vi "Differential Pressure Release Valve Test DAA.vi"(8 "error in (no error)":errorcluster, 10 "Model in":refnum<class "Model.lvclass">, 11 "Test Actuator State in":refnum<class "Test Actuator State.lvclass">) -> (0 "error out":errorcluster, 1 "Pass":bool, 2 "Model out":refnum<class "Model.lvclass">, 3 "Test Actuator State out":refnum<class "Test Actuator State.lvclass">)   [LabVIEW 2016, in "Test Actuator State.lvclass"]
uses:
  Test Actuator State.lvclass
  Model/Model/Model.lvclass
  Model/Model/Model.lvclass/Model.ctl
  Typedefs/ActuatorSetPoints.ctl
  <vilib>/Platform/TimedLoop/XDataNode/timing_clust.ctl
  <vilib>/Platform/TimedLoop/XDataNode/nitl_modes.ctl
  <vilib>/Platform/TimedLoop/XDataNode/wakeup.ctl
  <vilib>/platform/TimedLoop/XDataNode/XDataNode.xnode
  Typedefs/FAMT Typedefs.lvlib
  <vilib>/Platform/TimedLoop/XDataNode/XDNodeRunTimeDep.lvlib
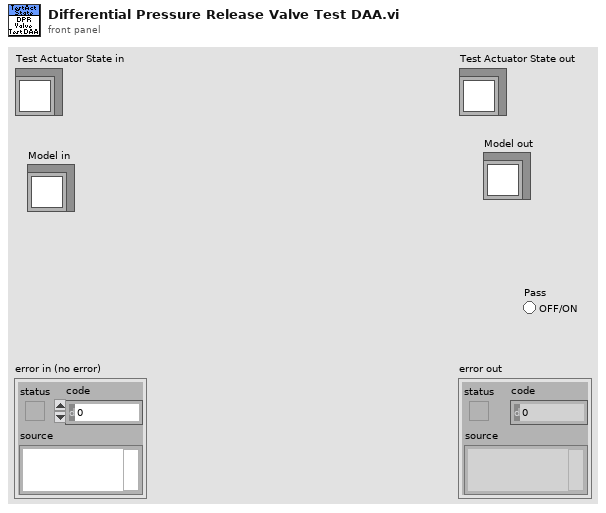
[diagram p1: front panel]
types:
  T1 = typedef "FAMT Typedefs.lvlib/DifferentialPressureReleaseValveTestSettings.ctl" = cluster{"Max Over Force (N)":dbl, "Process Time (s)":dbl, "Sample Time (s)":dbl}
  T2 = typedef "FAMT Typedefs.lvlib/ForcePair.ctl" = cluster{"Axial Force":dbl, "Lateral Force":dbl}
  T3 = typedef "FAMT Typedefs.lvlib/FullForceScanSettings.ctl" = cluster{"Force Tolerance (N)":dbl, "DAA Force Set Points":T2[], "Process Time (s)":dbl, "Sample Time (s)":dbl, "SAA Force Set Points":T2[]}
  T4 = cluster{"Top Left":T2, "Top Right":T2, "Bottom Right":T2, "Bottom Left":T2}
  T5 = typedef "FAMT Typedefs.lvlib/ActuatorSetPoints.ctl" = cluster{"Axial Force":dbl, "Lateral Force":dbl, "FC1 Force":dbl, "FC2 Force":dbl}
  T6 = typedef "XDNodeRunTimeDep.lvlib/timing_clust.ctl" = cluster{"Expected End [f-1]":u64, "Actual End [f-1]":u64, "Finished Late? [f-1]":bool, "Expected End [i-1]":u64, "Actual End [i-1]":u64, "Finished Late? [i-1]":bool, "Expected Start [i]":u64, "Actual Start [i]":u64, "Expected Start [f]":u64, "Actual Start [f]":u64, "Source Name":string, "Structure Name":string, "Period":i64, "Deadline":i64, "Offset":i64, "Start":i64, "Priority":i32, "Timeout":i32, "Mode":T7, "Wakeup Reason":T8, "Error":errorcluster, "Source Type":string, "Secondary Source Type":string, "Global End Time":u64, "Global Start Time":u64, "Frame Duration":u64, "Iteration Duration":u64, "Assigned CPU":i32, "I/O Scan Engine Mode":u32}
  T7 = typedef "XDNodeRunTimeDep.lvlib/nitl_modes.ctl" = enum32{"No Change", "Process missed periods, maintain original phase", "Discard missed periods, maintain original phase", "Process missed periods, ignore original phase", "Discard missed periods, ignore original phase"}
  T8 = typedef "XDNodeRunTimeDep.lvlib/wakeup.ctl" = enum32{"Normal", "Aborted", "Asynchronous wakeup", "Timing source error", "Timed loop error", "Timeout"}
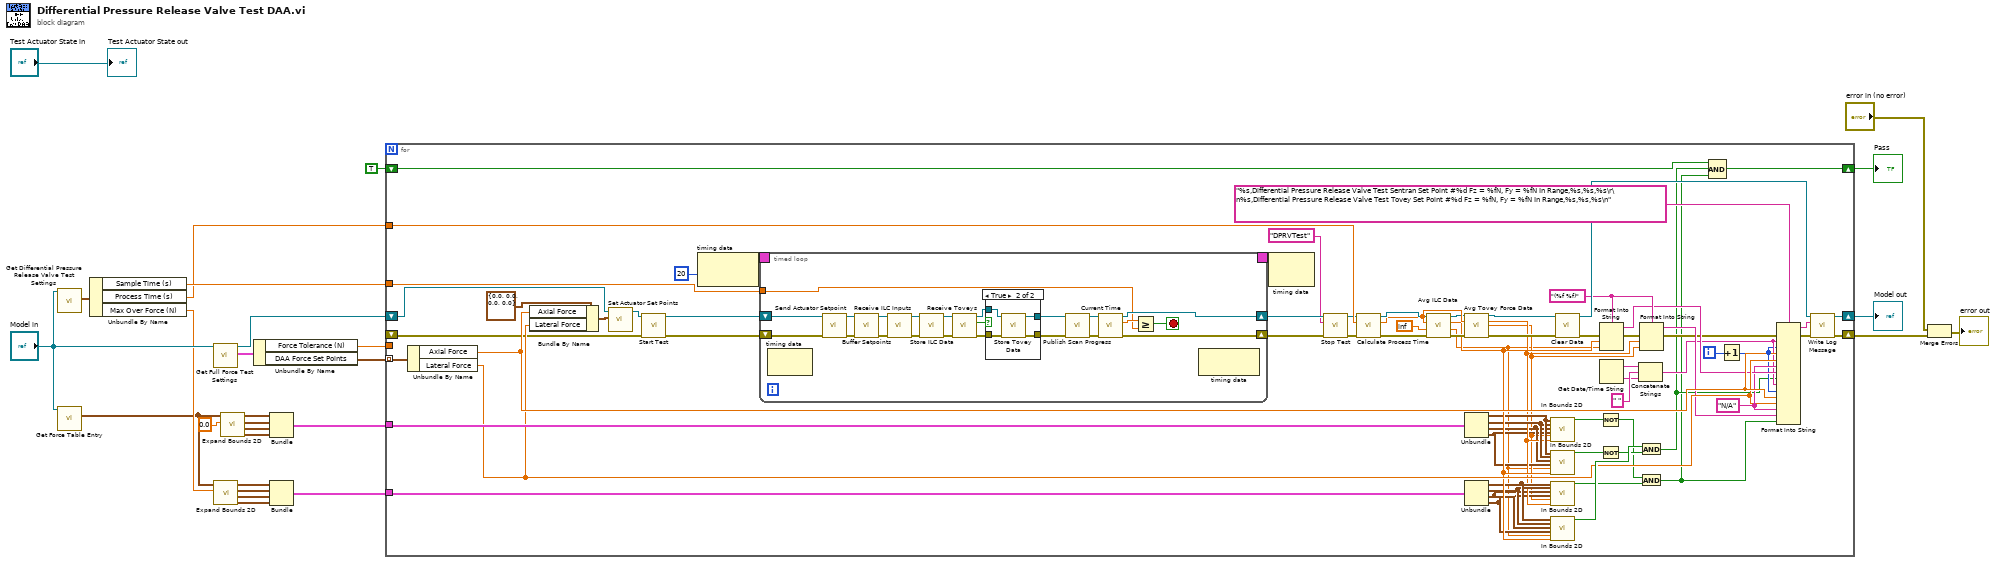
[diagram p0: block diagram]
diagram:
  n1 = call-dynamic "Get Differential Pressure Release Valve Test Settings.vi"("Model in"="Model in") -> ("Differential Pressure Release Valve Test Settings"=w18:T1)  [unwired: 9 in, 1 out]
  n2 = call "Get Force Table Entry.vi"("Model in"="Model in") -> ("Entry"=w10:T2[])  [unwired: 8 in, 2 out]
  n3 = Unbundle By Name(w18) -> ("Sample Time (s)"=w26:dbl, "Process Time (s)"=w25:dbl, "Max Over Force (N)"=w17:dbl)
  n4 = call "Get Full Force Test Settings.vi"("Model in"="Model in") -> ("Full Force Test Settings"=w20:T3, "Model out"=w27:refnum<class "Model.lvclass">)  [unwired: 9 in]
  n5 = call "Expand Bounds 2D.vi"("Tolerance (N)"=w17, "Entry"=w10) -> ("Bottom Left"=w12:T2, "Bottom Right"=w13:T2, "Top Right"=w14:T2, "Top Left"=w15:T2)  [unwired: 6 in]
  n6 = call "Expand Bounds 2D.vi"("Tolerance (N)"=0.0, "Entry"=w10) -> ("Bottom Left"=w5:T2, "Bottom Right"=w6:T2, "Top Right"=w7:T2, "Top Left"=w8:T2)  [unwired: 6 in]
  n7 = Unbundle By Name(w20) -> ("Force Tolerance (N)"=w3:dbl, "DAA Force Set Points"=w16:T2[])
  n8 = Bundle("Top Left"=w8, "Top Right"=w7, "Bottom Right"=w6, "Bottom Left"=w5) -> (w4:T4)  [unwired: 1 in]
  n9 = Bundle("Top Left"=w15, "Top Right"=w14, "Bottom Right"=w13, "Bottom Left"=w12) -> (w11:T4)  [unwired: 1 in]
  n10 = for {
    tunnel: w16 -> [w91] mode=indexing
    shift-right: [w95] -> w22
    shift-left: w27 -> [w98]
    tunnel: w26 -> [w97]
    tunnel: w25 -> [w87]
    shift-right: [w88] -> w21
    shift-left: _ -> [w44]
    tunnel: w11 -> [w80]
    tunnel: w4 -> [w79]
    tunnel: w3 -> [_]
    shift-right: [w29] -> w1
    shift-left: TRUE -> [w32]
    i -> [w93]
    w69 = "N/A" ("input 5")
    w73 = "(%f %f)" ("format string")
    n11 = Unbundle By Name(w91) -> ("Axial Force"=w75:dbl, "Lateral Force"=w74:dbl)
    n12 = Bundle By Name(cluster=T5 {"Axial Force"=0.0, "Lateral Force"=0.0, "FC1 Force"=0.0, "FC2 Force"=0.0} ("Actuator Set Points"), "Axial Force"=w75, "Lateral Force"=w74) -> (w92:T5)
    n13 = call "Set Actuator Set Points.vi"("Actuator Set Points"=w92, "Model in"=w98) -> ("Model out"=w46:refnum<class "Model.lvclass">)  [unwired: 9 in]
    n14 = call "Start Test.vi"("error in (no error)"=w44, "Model in"=w46) -> ("error out"=w43:errorcluster, "Model out"=w45:refnum<class "Model.lvclass">)  [unwired: 8 in]
    n15 = node-c288(i64 20 ("Period")) -> (w49:T6)
    n16 = timed-loop {
      shift-right: [w117] -> w42
      shift-left: w45 -> [w121]
      shift-right: [w116] -> w40
      shift-left: w43 -> [w119]
      tunnel: w97 -> [w114]
      timing: w49 -> [_]
      timing-out: [_] -> w48
      stop <- w113 stop-if-true
      n17 = node-c288() -> ()  [unwired: 1 in, 1 out]
      n18 = call "Send Actuator Setpoint.vi"("error in (no error)"=w119, "Model in"=w121) -> ("error out"=w101:errorcluster, "Model out"=w103:refnum<class "Model.lvclass">)  [unwired: 8 in]
      n19 = call "Buffer Setpoints.vi"("error in (no error)"=w101, "Model in"=w103) -> ("error out"=w100:errorcluster, "Model out"=w102:refnum<class "Model.lvclass">)  [unwired: 8 in]
      n20 = call "Receive ILC Inputs.vi"("error in (no error)"=w100, "Model in"=w102) -> ("error out"=w118:errorcluster, "Model out"=w120:refnum<class "Model.lvclass">)  [unwired: 8 in]
      n21 = call "Store ILC Data.vi"("error in (no error)"=w118, "Model in"=w120) -> ("error out"=w111:errorcluster, "Model out"=w112:refnum<class "Model.lvclass">)  [unwired: 8 in]
      n22 = call "Receive Toveys.vi"("error in (no error)"=w111, "Model in"=w112) -> ("error out"=w109:errorcluster, "Data Received"=w108:bool, "Model out"=w110:refnum<class "Model.lvclass">)  [unwired: 7 in]
      n23 = case shown="True" w108 {
        tunnel: w110 -> [w125 w129]
        tunnel: w109 -> [w124 w128]
        tunnel: [w124 w127] -> w104
        tunnel: [w125 w126] -> w107
        frame False {
        }
        frame True {
          n24 = call "Store Tovey Data.vi"("error in (no error)"=w128, "Model in"=w129) -> ("error out"=w127:errorcluster, "Model out"=w126:refnum<class "Model.lvclass">)  [unwired: 8 in]
        }
      }
      n25 = call "Publish Scan Progress.vi"("error in (no error)"=w104, "Model in"=w107) -> ("error out"=w105:errorcluster, "Model out"=w106:refnum<class "Model.lvclass">)  [unwired: 8 in]
      n26 = call "Current Time.vi"("error in (no error)"=w105, "Model in"=w106) -> ("error out"=w116:errorcluster, "Time"=w115:dbl, "Model out"=w117:refnum<class "Model.lvclass">)  [unwired: 7 in]
      n27 = Greater Or Equal?(x=w115, y=w114) -> (x >= y?=w113:bool)
      n28 = node-c288() -> ()  [unwired: 1 in, 1 out]
    }
    n29 = node-c288(w48) -> ()  [unwired: 1 out]
    n30 = call "Stop Test.vi"("error in (no error)"=w40, "Test"="DPRVTest", "Model in"=w42) -> ("error out"=w39:errorcluster, "Model out"=w41:refnum<class "Model.lvclass">)  [unwired: 7 in]
    n31 = call "Calculate Process Time.vi"("error in (no error)"=w39, "Seconds"=w87, "Model in"=w41) -> ("error out"=w85:errorcluster, "Time"=w84:dbl, "Model out"=w86:refnum<class "Model.lvclass">)  [unwired: 6 in]
    n32 = call "Avg ILC Data.vi"("error in (no error)"=w85, "Before This Time"=inf, "After This Time"=w84, "Model in"=w86) -> ("error out"=w83:errorcluster, "Fy"=w51:dbl, "Fz"=w72:dbl, "Model out"=w60:refnum<class "Model.lvclass">)  [unwired: 4 in]
    n33 = call "Avg Tovey Force Data.vi"("Model in"=w60, "After This Time"=w84, "error in (no error)"=w83) -> ("Model out"=w82:refnum<class "Model.lvclass">, "Fz"=w64:dbl, "Fy"=w52:dbl, "error out"=w81:errorcluster)  [unwired: 8 in, 1 out]
    n34 = Unbundle(w79) -> ("Top Left"=w66:T2, "Top Right"=w65:T2, "Bottom Right"=w54:T2, "Bottom Left"=w53:T2)
    n35 = Unbundle(w80) -> ("Top Left"=w68:T2, "Top Right"=w67:T2, "Bottom Right"=w56:T2, "Bottom Left"=w55:T2)
    n36 = call "In Bounds 2D.vi"("Top Left"=w66, "Top Right"=w65, "Bottom Right"=w54, "Bottom Left"=w53, "Lateral"=w52, "Axial"=w64) -> ("InBounds"=w63:bool)  [unwired: 13 in]
    n37 = call "In Bounds 2D.vi"("Top Left"=w66, "Top Right"=w65, "Bottom Right"=w54, "Bottom Left"=w53, "Lateral"=w51, "Axial"=w72) -> ("InBounds"=w78:bool)  [unwired: 13 in]
    n38 = call "In Bounds 2D.vi"("Top Left"=w68, "Top Right"=w67, "Bottom Right"=w56, "Bottom Left"=w55, "Lateral"=w52, "Axial"=w64) -> ("InBounds"=w61:bool)  [unwired: 13 in]
    n39 = call "In Bounds 2D.vi"("Top Left"=w68, "Top Right"=w67, "Bottom Right"=w56, "Bottom Left"=w55, "Lateral"=w51, "Axial"=w72) -> ("InBounds"=w77:bool)  [unwired: 13 in]
    n40 = call "Clear Data.vi"("error in (no error)"=w81, "Model in"=w82) -> ("error out"=w59:errorcluster, "Model out"=w96:refnum<class "Model.lvclass">)  [unwired: 8 in]
    n41 = Not(x=w63) -> (.not. x?=w62:bool)
    n42 = Not(x=w78) -> (.not. x?=w76:bool)
    n43 = Format Into String(format string=w73, error in=w59, w72, w51) -> (resulting string=w71:string, error out=w58:errorcluster)  [unwired: 1 in]
    n44 = Get Date/Time String() -> (date string=w35:string, time string=w36:string)  [unwired: 3 in]
    n45 = Concatenate Strings(w35, " " ("string"), w36) -> (w34:string)
    n46 = Format Into String(format string=w73, error in=w58, w64, w52) -> (resulting string=w70:string, error out=w57:errorcluster)  [unwired: 1 in]
    n47 = And(x=w77, y=w76) -> (x .and. y?=w31:bool)
    n48 = And(x=w62, y=w61) -> (x .and. y?=w30:bool)
    n49 = Compound Arithmetic op=AND(w32, w31, w30) -> (w29:bool)
    n50 = Increment(x=w93) -> (x+1=w33:i32)
    n51 = Format Into String(format string="%s,Differential Pressure Release Valve Test Sentran Set Point #%d Fz = %fN, Fy = %fN In Range,%s,%s,%s\r\n%s,Differential Pressure Release Valve Test Tovey Set Point #%d Fz = %fN, Fy = %fN In Range,%s,%s,%s\n", error in=w57, w34, w33, w75, w74, w69, w71, w31, w34, w33, w75, w74, w69, w70, w30) -> (resulting string=w90:string, error out=w89:errorcluster)  [unwired: 1 in]
    n52 = call "Write Log Message.vi"("error in (no error)"=w89, "Message"=w90, "Model in"=w96) -> ("error out"=w88:errorcluster, "Model out"=w95:refnum<class "Model.lvclass">)  [unwired: 7 in]
  }
  "Model out" <- w22
  "Pass" <- w1
  n53 = Merge Errors("error in (no error)", w21) -> (→"error out":errorcluster)
  "Test Actuator State out" <- "Test Actuator State in"
